vi "End.vi"(8 "error in (no error)":errorcluster, 11 "SPARC4_GUI in":refnum<class "SPARC4_GUI.lvclass">) -> (0 "error out":errorcluster, 3 "SPARC4_GUI out":refnum<class "SPARC4_GUI.lvclass">)   [LabVIEW 2018, in "SPARC4_GUI.lvclass"]
uses:
  SPARC4_GUI.lvclass
  SPARC4_GUI.lvclass/SPARC4_GUI.ctl
  Stream/Stream.lvclass
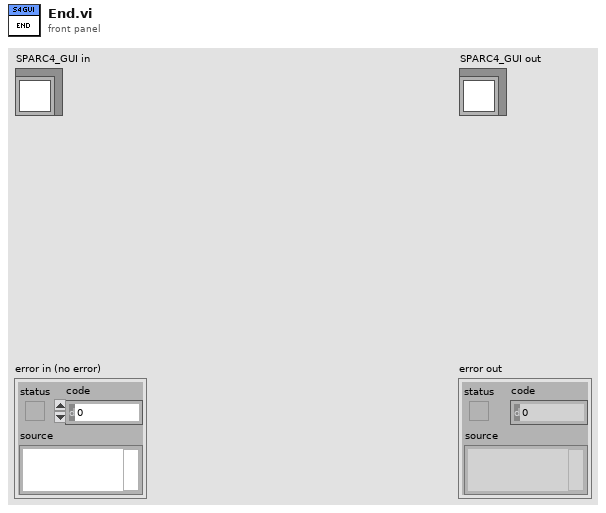
[diagram p1: front panel]
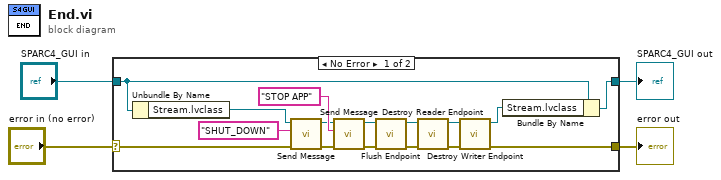
[diagram p0: block diagram]
diagram:
  n1 = case shown="No Error" "error in (no error)" {
    selector: "error in (no error)" -> [w7 w22]
    tunnel: [w13 w22] -> w3
    tunnel: [w11 w21] -> w1
    tunnel: "SPARC4_GUI in" -> [w12 w21]
    frame No Error {
      n2 = Unbundle By Name(w12) -> ("Stream.lvclass"=w6:refnum<class "Stream.lvclass">)
      n3 = call "Send Message.vi"("error in (no error)"=w7, "Message"="SHUT_DOWN", "Stream in"=w6) -> ("error out"=w8:errorcluster, "Stream out"=w9:refnum<class "Stream.lvclass">)  [unwired: 7 in]
      n4 = call "Send Message.vi"("error in (no error)"=w8, "Message"="STOP APP", "Stream in"=w9) -> ("error out"=w20:errorcluster, "Stream out"=w19:refnum<class "Stream.lvclass">)  [unwired: 7 in]
      n5 = call "Flush Endpoint.vi"("error in (no error)"=w20, "Stream in"=w19) -> ("error out"=w16:errorcluster, "Stream out"=w17:refnum<class "Stream.lvclass">)  [unwired: 8 in]
      n6 = call "Destroy Reader Endpoint.vi"("error in (no error)"=w16, "Stream in"=w17) -> ("error out"=w15:errorcluster, "Stream out"=w14:refnum<class "Stream.lvclass">)  [unwired: 8 in]
      n7 = call "Destroy Writer Endpoint.vi"("error in (no error)"=w15, "Stream in"=w14) -> ("error out"=w13:errorcluster, "Stream out"=w10:refnum<class "Stream.lvclass">)  [unwired: 8 in]
      n8 = Bundle By Name(cluster=w12, "Stream.lvclass"=w10) -> (w11:refnum<class "SPARC4_GUI.lvclass">)
    }
    frame Error {
    }
  }
  "error out" <- w3
  "SPARC4_GUI out" <- w1
